vi "Dead Zone.vi"(4 "Dead Zone limit":dbl=0.2, 7 "Rotate":dbl format="%#_13g", 8 "TranslateY":dbl format="%#_13g", 9 "TranslateX":dbl format="%#_13g") -> (1 "Rotate":dbl, 2 "TranslateY":dbl, 3 "TranslateX":dbl)   [LabVIEW 2014]
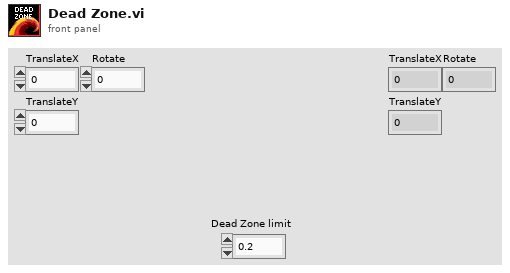
[diagram p1: front panel]
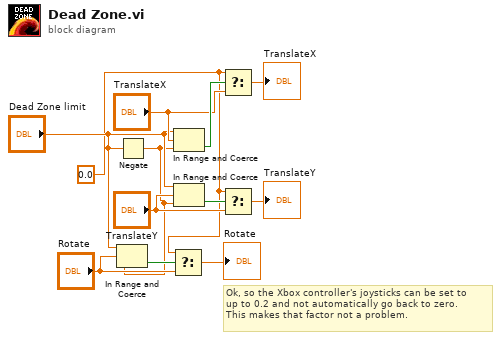
[diagram p0: block diagram]
diagram:
  w1 = 0.0 ("t")
  # "Ok, so the Xbox controller's joysticks can be set to \nup to 0.2 and not automatically go back to zero.\nThis makes that factor not a problem."
  n1 = Negate(x="Dead Zone limit") -> (-x=w2:dbl)
  n2 = In Range and Coerce(upper limit="Dead Zone limit", x="Rotate", lower limit=w2) -> (In Range?=w6:bool)  [unwired: 1 out]
  n3 = Select(t=w1, s=w6, f="Rotate") -> (s? t:f=→"Rotate":dbl)
  n4 = In Range and Coerce(upper limit="Dead Zone limit", x="TranslateX", lower limit=w2) -> (In Range?=w12:bool)  [unwired: 1 out]
  n5 = In Range and Coerce(upper limit="Dead Zone limit", x="TranslateY", lower limit=w2) -> (In Range?=w11:bool)  [unwired: 1 out]
  n6 = Select(t=w1, s=w12, f="TranslateX") -> (s? t:f=→"TranslateX":dbl)
  n7 = Select(t=w1, s=w11, f="TranslateY") -> (s? t:f=→"TranslateY":dbl)
